vi "SendUserEventMessage.vi"(5 "atributes":variant, 7 "urgent? (F)":bool, 8 "error in":errorcluster, 9 "data":variant, 10 "name":string, 11 "message ref in":refnum<class "CLM_LocalMessage_UserEvent.lvclass">) -> (0 "error out":errorcluster, 3 "message ref out":refnum<class "CLM_LocalMessage_UserEvent.lvclass">)   [LabVIEW 2013, in "CLM_LocalMessage_UserEvent.lvclass"]
uses:
  CLM_LocalMessage_UserEvent.lvclass
  CLM_LocalMessage_UserEvent.lvclass/CLM_LocalMessage_UserEvent.ctl
  LocalMessage/CLM_LocalMessage.lvclass
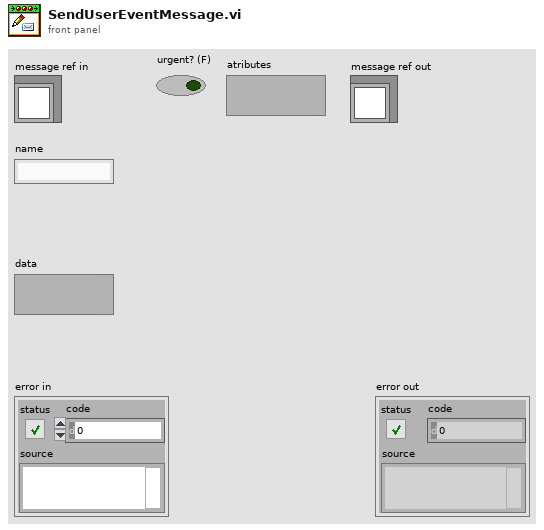
[diagram p1: front panel]
types:
  T1 = typedef "CLM_LocalMessage.lvclass/Message.ctl" = cluster{"name":string, "data":variant, "attributes":variant, "urgent":bool}
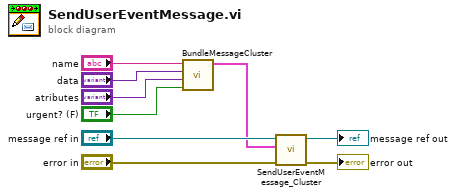
[diagram p0: block diagram]
diagram:
  n1 = call "BundleMessageCluster.vi"("urgent? (F)"="urgent? (F)", "atributes"="atributes", "data"="data", "name"="name") -> ("message"=w2:T1)  [unwired: 7 in]
  n2 = call "SendUserEventMessage_Cluster.vi"("error in"="error in", "message"=w2, "message ref in"="message ref in") -> ("error out"=→"error out":errorcluster, "message ref out"=→"message ref out":refnum<class "CLM_LocalMessage_UserEvent.lvclass">)  [unwired: 7 in]
